vi "Stop Core.vi"(10 "final error code":i32, 11 "CS++DeviceActor in":refnum<class "CS++DeviceActor.lvclass">) -> (3 "CS++DeviceActor out":refnum<class "CS++DeviceActor.lvclass">)   [LabVIEW 2014, in "CS++DeviceActor.lvlib" / "CS++DeviceActor.lvclass"]
doc: "(<B>Filename</B>: Actor Framework.lvlib:Actor.lvclass:Stop Core.vi)\n\nDefines what the actor does before it stops. Use the <B>final error code</B> input to determine whether the actor shut down in response to an error.\n\nBy default, this method does nothing. A descendant class may override it to define behavior, such as shutting down any processes the actor initiated in its override of the Actor Core method."
uses:
  CS++DeviceActor.lvclass
  CS++DeviceActor.lvclass/CS++DeviceActor.ctl
  CS++BaseActor/CS++BaseActor.lvclass
  Classes/CS++ProcessVariables/PVConnection/PVConnection.lvclass
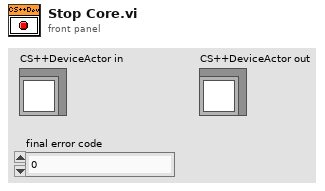
[diagram p1: front panel]
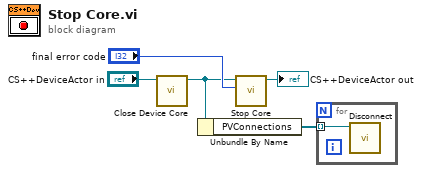
[diagram p0: block diagram]
diagram:
  n1 = call-dynamic "Close Device Core.vi"("CS++DeviceActor in"="CS++DeviceActor in") -> ("CS++DeviceActor out"=w2:refnum<class "CS++DeviceActor.lvclass">)  [unwired: 9 in, 1 out]
  n2 = Unbundle By Name(w2) -> ("PVConnections"=w1:refnum<class "PVConnection.lvclass">[])
  n3 = call-parent "Stop Core.vi"("final error code"="final error code", "CS++BaseActor in"=w2) -> ("CS++BaseActor out"=→"CS++DeviceActor out":refnum<class "CS++DeviceActor.lvclass">)  [unwired: 9 in]
  n4 = for {
    tunnel: w1 -> [w6] mode=indexing
    n5 = call-dynamic "Disconnect.vi"("PVConnection in"=w6) -> ()  [unwired: 9 in, 2 out]
  }
